vi "PH_Cam_BaseClass.Save Img Proc.vi"(0 "VI in":refnum<vi>, 5 "error in (no error)":errorcluster) -> (14 "VI out":refnum<vi>, 19 "error out":errorcluster)   [LabVIEW 2014, in "PH_Cam_BaseClass.lvlib"]
uses:
  PH_Cam_BaseClass.lvlib
  PH_Common/Names/PH_Names.File Types.ctl
  PH_Common/PH_Common.lvlib
  CS_Core/CSSystem/CSSystemLib/CSSystemLib.lvlib
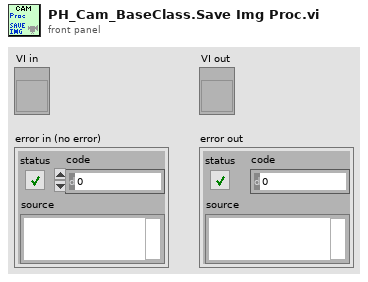
[diagram p1: front panel]
types:
  T1 = enum16{"Left Button", "Center Button", "Right Button", "Window Close"}
  T2 = typedef "PH_Common.lvlib/PH_Names.File Types.ctl" = string
  T3 = enum16{"open", "open or create", "create or replace", "create", "open (read only)"}
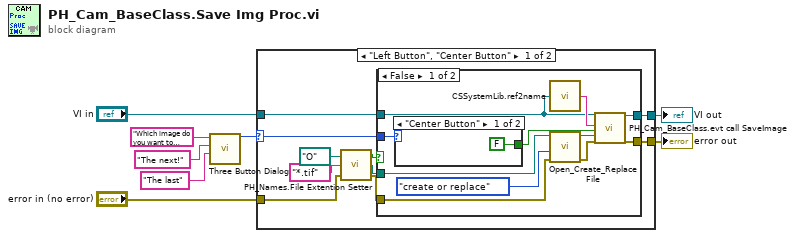
[diagram p0: block diagram]
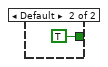
[diagram p2: hidden frame]
diagram:
  n1 = call <vilib>:"Three Button Dialog.vi"("Center Button Text (\"No\")"="The last" ("Center Button Text (\"No\")"), "Left Button Text (\"Yes\")"="The next!" ("Left Button Text (\"Yes\")"), "message"="Which image do you want to save?") -> ("Which Button?"=w8:T1)  [unwired: 8 in]
  n2 = case shown="\"Left Button\", \"Center Button\"" w8 {
    selector: w8 -> [w11 _]
    tunnel: "error in (no error)" -> [w10 w34]
    tunnel: [w16 w34] -> w2
    tunnel: [w17 w35] -> w3
    tunnel: "VI in" -> [w18 w35]
    frame "Left Button", "Center Button" {
      n3 = call "PH_Names.File Extention Setter.vi"("error in (no error)"=w10, "File Type"=T2 "*.tif" ("file name extinction"), "start path (O:\\)"=path "O:/" ("start path (O:\\)")) -> ("error out"=w9:errorcluster, "path with extension"=w14:path, "cancelled?"=w13:bool)
      n4 = case shown="False" w13 {
        tunnel: w18 -> [w19 w33]
        tunnel: [w29 w33] -> w17
        tunnel: [w28 w32] -> w16
        tunnel: w9 -> [w27 w32]
        tunnel: w14 -> [w24 _]
        tunnel: w11 -> [w22 _]
        frame False {
          n5 = case shown="\"Center Button\"" w22 {
            tunnel: [FALSE ("Next/Last (Next)") TRUE ("Next/Last (Next)")] -> w23
            frame "Center Button" {
            }
            frame Default {
            }
          }
          n6 = call "CSSystemLib.ref2name.vi"("obj refnum"=w19) -> ("name"=w20:string)
          n7 = call <vilib>:"Open_Create_Replace File.vi"("error in (no error)"=w27, "function (open:0)"=T3."create or replace", "file path"=w24) -> ("error out"=w26:errorcluster, "refnum"=w25:refnum<file>)  [unwired: 5 in, 2 out]
          n8 = call "PH_Cam_BaseClass.evt call SaveImage.vi"("i ref in"=w19, "Instance"=w20, "Last/Next"=w23, "File refnum"=w25, "error in (no error)"=w26) -> ("i ref out"=w29:refnum<vi>, "error out"=w28:errorcluster)  [unwired: 13 in]
        }
        frame True {
        }
      }
    }
    frame Default {
    }
  }
  "VI out" <- w3
  "error out" <- w2
